vi "LatchingActionOnArray.vi"(11 "Array of booleans":bool[](array[boolean])) -> (3 "Latched booleeans":bool[](array[boolean]))   [LabVIEW 2014]
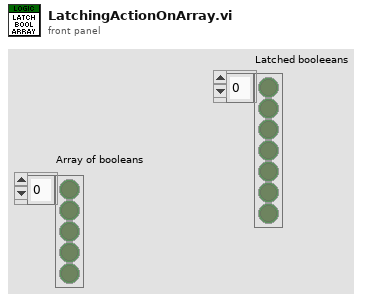
[diagram p1: front panel]
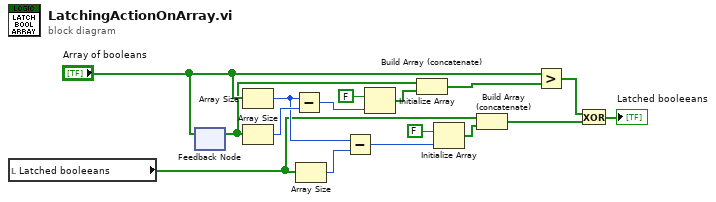
[diagram p0: block diagram]
diagram:
  n1 = local read "Latched booleeans"() -> (w2:bool[])
  n2 = feedback-in #1("Array of booleans") -> ()
  n3 = feedback #1() -> (w9:bool[])  [unwired: 1 in]
  n4 = Array Size(array="Array of booleans") -> (size(s)=w3:i32)
  n5 = Array Size(array=w9) -> (size(s)=w13:i32)
  n6 = Subtract(x=w3, y=w13) -> (x-y=w12:i32)
  n7 = Array Size(array=w2) -> (size(s)=w4:i32)
  n8 = Subtract(x=w3, y=w4) -> (x-y=w5:i32)
  n9 = Initialize Array(FALSE, w12) -> (w10:bool[])
  n10 = Build Array (concatenate)(w9, w10) -> (w8:bool[])
  n11 = Initialize Array(FALSE, w5) -> (w7:bool[])
  n12 = Build Array (concatenate)(w2, w7) -> (w1:bool[])
  n13 = Greater?(x="Array of booleans", y=w8) -> (0:w15:bool[])
  n14 = Exclusive Or(1:w1, 2:w15) -> (0:→"Latched booleeans":bool[])
